vi "Initialize Timings Arrays.vi"(8 "error in (no error)":errorcluster, 11 "Readout Charact in":refnum<class "Readout Charact.lvclass">) -> (0 "error out":errorcluster, 3 "Readout Charact out":refnum<class "Readout Charact.lvclass">)   [LabVIEW 2018, in "Readout Charact.lvclass"]
uses:
  Readout Charact.lvclass
  Readout Charact.lvclass/Readout Charact.ctl
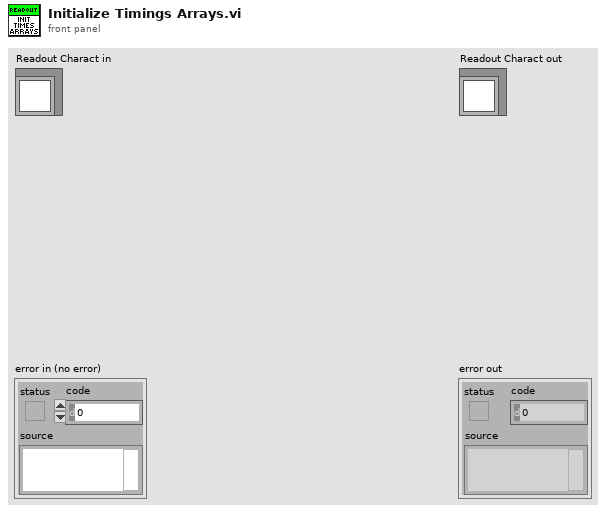
[diagram p1: front panel]
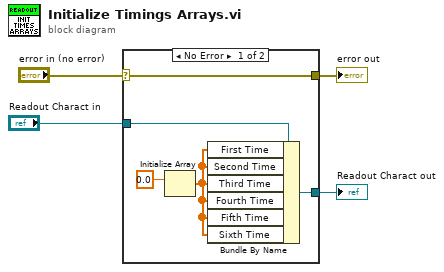
[diagram p0: block diagram]
diagram:
  n1 = case shown="No Error" "error in (no error)" {
    selector: "error in (no error)" -> [w9 w11]
    tunnel: [w9 w11] -> w3
    tunnel: [w7 w10] -> w1
    tunnel: "Readout Charact in" -> [w8 w10]
    frame No Error {
      n2 = Initialize Array(0.0) -> (w5:dbl[])  [unwired: 1 in]
      n3 = Bundle By Name(cluster=w8, "First Time"=w5, "Second Time"=w5, "Third Time"=w5, "Fourth Time"=w5, "Fifth Time"=w5, "Sixth Time"=w5) -> (w7:refnum<class "Readout Charact.lvclass">)
    }
    frame Error {
    }
  }
  "error out" <- w3
  "Readout Charact out" <- w1
